vi "XOR Truth Table.vi"() -> ()   [LabVIEW 2016]
panel:
  out "A xor B":bool[](array[boolean])=[FALSE, TRUE, TRUE, FALSE]
  in  "B":bool[](array[boolean])=[FALSE, TRUE, FALSE, TRUE]
  in  "A":bool[](array[boolean])=[FALSE, FALSE, TRUE, TRUE]
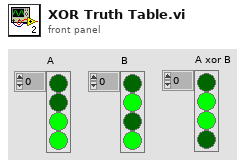
[diagram p1: front panel]
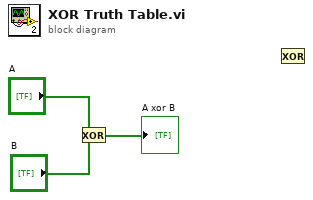
[diagram p0: block diagram]
diagram:
  n1 = Exclusive Or(1:"B", 2:"A") -> (0:→"A xor B":bool[])
  n2 = Exclusive Or() -> ()  [unwired: 2 in, 1 out]
